vi "avg.vi"(1 "Array":dbl[](array[numeric]) format="%.2f") -> (0 "Numeric":dbl format="%.2f")   [LabVIEW 2010]
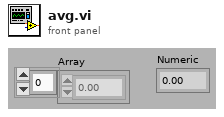
[diagram p1: front panel]
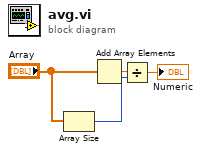
[diagram p0: block diagram]
diagram:
  n1 = Array Size(array="Array") -> (size(s)=w1:i32)
  n2 = Add Array Elements(numeric array="Array") -> (sum=w3:dbl)
  n3 = Divide(x=w3, y=w1) -> (x/y=→"Numeric":dbl)
